vi "Dispose Screen.vi"(8 "error in (no error)":errorcluster caption="错误输入（无错误）", 11 "Screen 输入":refnum<class "Screen.lvclass"> caption="DNL_LabVIEW Object in") -> (0 "error out":errorcluster caption="错误输出", 3 "Screen 输出":refnum<class "Screen.lvclass"> caption="DNL_LabVIEW Object out")   [LabVIEW 2011, in "Screen.lvclass"]
uses:
  Screen.lvclass
  Screen.lvclass/Screen.ctl
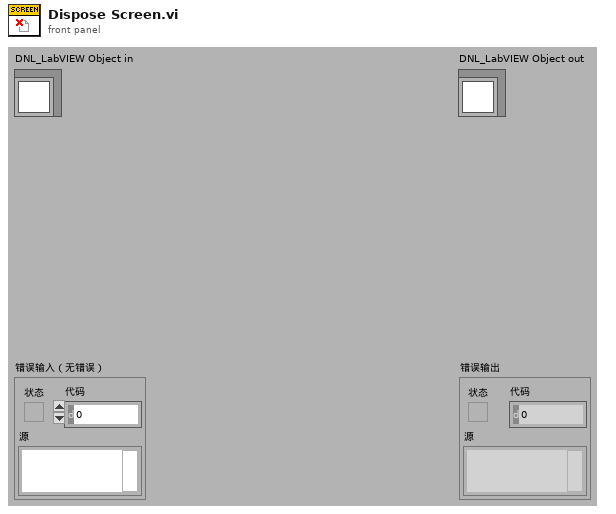
[diagram p1: front panel]
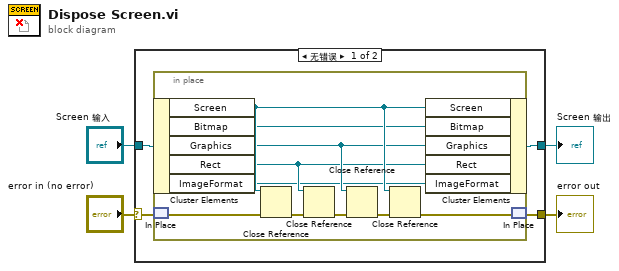
[diagram p0: block diagram]
diagram:
  n1 = case shown="无错误" "error in (no error)" {
    selector: "error in (no error)" -> [w7 w19]
    tunnel: [w5 w20] -> w2
    tunnel: "Screen 输入" -> [w8 w20]
    tunnel: [w6 w19] -> w1
    frame No Error {
      n2 = in-place {
        n3 = in-place-cluster #1(w8) -> ("Screen"=w17:refnum<k24>, "Bitmap"=w12:refnum<k24>, "Graphics"=w11:refnum<k24>, "Rect"=w10:refnum<k24>, "ImageFormat"=w9:refnum<k24>)
        n4 = in-place-match #2(w7) -> (w18:errorcluster)
        n5 = Close Reference(reference=w17, error in (no error)=w18) -> (error out=w16:errorcluster)
        n6 = Close Reference(reference=w10, error in (no error)=w16) -> (error out=w15:errorcluster)
        n7 = Close Reference(reference=w11, error in (no error)=w15) -> (error out=w14:errorcluster)
        n8 = Close Reference(reference=w17, error in (no error)=w14) -> (error out=w13:errorcluster)
        n9 = in-place-cluster #1("Screen"=w17, "Bitmap"=w12, "Graphics"=w11, "Rect"=w10, "ImageFormat"=w9) -> (w5:refnum<class "Screen.lvclass">)
        n10 = in-place-match #2(w13) -> (w6:errorcluster)
      }
    }
    frame Error {
    }
  }
  "error out" <- w1
  "Screen 输出" <- w2
